vi "V3fit.vi"(3 "output control":T2, 4 "data":T1, 5 "X":dbl[](array[numeric]), 6 "a":dbl[](array[numeric])) -> (0 "error out":errorcluster, 1 "f'(X,a)":dbl[][](array[numeric]), 2 "f(X,a)":dbl[](array[numeric]))   [LabVIEW 2018]
doc: "This template is the starting point for creating a model function to be passed to the Nonlinear Curve Fit.vi."
uses:
  <vilib>/gmath/NumericalOptimization/LM_output select.ctl
  <vilib>/gmath/NumericalOptimization/objective function data.ctl
  <vilib>/gmath/NI_Gmath.lvlib
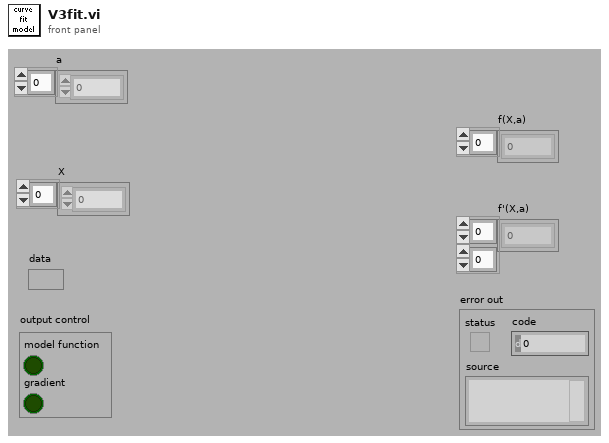
[diagram p1: front panel]
types:
  T1 = typedef "NI_Gmath.lvlib/objective function data.ctl" = variant
  T2 = typedef "NI_Gmath.lvlib/LM_output select.ctl" = cluster{"model function":bool, "gradient":bool}
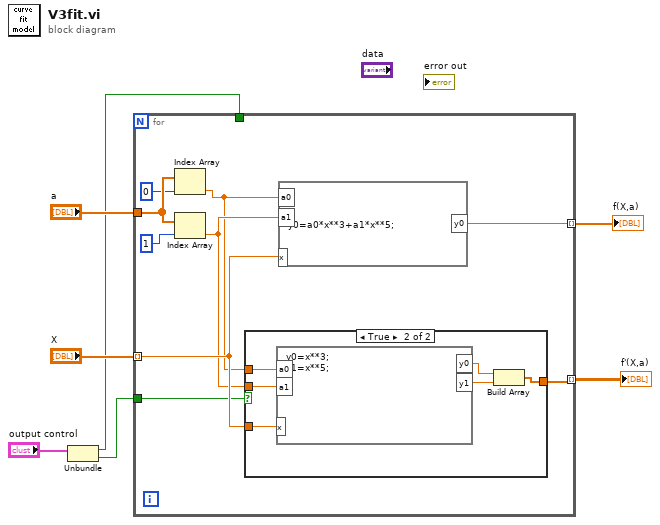
[diagram p0: block diagram]
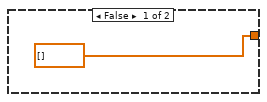
[diagram p2: hidden frame]
diagram:
  n1 = Unbundle("output control") -> ("model function"=w1:bool, "gradient"=w2:bool)
  n2 = for {
    tunnel: "a" -> [w14]
    tunnel: "X" -> [w16] mode=indexing
    tunnel: [w15] -> w5 mode=indexing
    tunnel: [w8] -> w4 mode=indexing
    tunnel: w2 -> [w9]
    tunnel: w1 -> [_]
    n3 = Index Array(array=w14, index=0) -> (element=w10:dbl)
    n4 = Index Array(array=w14, index=1) -> (element=w11:dbl)
    n5 = case shown="True" w9 {
      tunnel: w16 -> [_ w23]
      tunnel: w11 -> [_ w22]
      tunnel: w10 -> [_ w21]
      tunnel: [dbl[] [] w18] -> w8
      frame False {
      }
      frame True {
        n6 = formula code="y0=x**3;\ny1=x**5;"("x"=w23, "a0"=w21, "a1"=w22) -> ("y0"=w19:dbl, "y1"=w20:dbl)
        n7 = Build Array(w19, w20) -> (w18:dbl[])
      }
    }
    n8 = formula code="y0=a0*x**3+a1*x**5;"("x"=w16, "a0"=w10, "a1"=w11) -> ("y0"=w15:dbl)
  }
  "f(X,a)" <- w5
  "f'(X,a)" <- w4
